vi "serial-read-mxp-board.vi"() -> ()   [LabVIEW 2018]
uses:
  bno055.ctl
  <vilib>/Rock Robotics/WPI/SerialPort/WPI_SerialPort.ctl
panel:
  out "BNO055":T1
  in  "stop":bool
  out "Read String":string
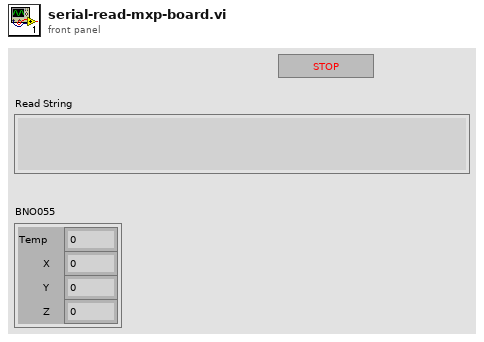
[diagram p1: front panel]
types:
  T1 = typedef "bno055.ctl" = cluster{"Temp":dbl, "X":dbl, "Y":dbl, "Z":dbl}
  T2 = typedef "WPI_SerialPort.ctl" = enum16{"Onboard RS-232", "MXP TTL", "USB 1", "USB 2"}
  T3 = typedef "WPI_SerialPortRef.ctl" = cluster{"DevStatus":errorcluster, "Serial Port Name":refnum<visa-resource-name>}
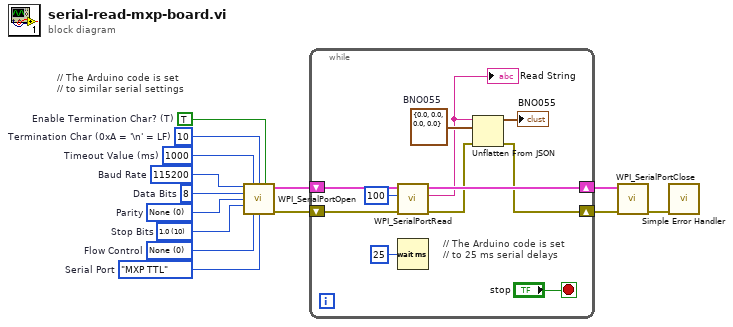
[diagram p0: block diagram]
diagram:
  w4 = WPI_SerialPort."MXP TTL"  # Serial Port
  w5 = u16 0 items=["None", "XON/XOFF", "RTS/CTS", "XON/XOFF & RTS/CTS", "DTR/DSR", "XON/XOFF & DTR/DSR"]  # Flow Control
  w6 = u16 10 items=["1.0"=10, "1.5"=15, "2.0"=20]  # Stop Bits
  w7 = u16 0 items=["None", "Odd", "Even", "Mark", "Space"]  # Parity
  w3 = u16 8  # Data Bits
  w8 = u32 115200  # Baud Rate
  w9 = u32 1000  # Timeout Value (ms)
  w10 = u8 10  # Termination Char (0xA = '\n' = LF)
  w11 = TRUE  # Enable Termination Char? (T)
  # "// The Arduino code is set \n// to similar serial settings"
  n1 = call <vilib>:"WPI_SerialPortOpen.vi"("Baud Rate"=w8, "Timeout Value (ms)"=w9, "Termination Char (0xA = '\\n' = LF)"=w10, "Enable Termination Char? (T)"=w11, "Data Bits"=w3, "Parity"=w7, "Stop Bits"=w6, "Flow Control"=w5, "Serial Port"=w4) -> ("SerialPortRef"=w2:T3, "error out"=w14:errorcluster)  [unwired: 5 in]
  n2 = while {
    shift-right: [w17] -> w13
    shift-left: w14 -> [w20]
    shift-right: [w25] -> w1
    shift-left: w2 -> [w21]
    stop <- "stop" stop-if-true
    w19 = T1 {"Temp"=0.0, "X"=0.0, "Y"=0.0, "Z"=0.0}  # BNO055
    # "// The Arduino code is set \n// to 25 ms serial delays"
    n3 = call <vilib>:"WPI_SerialPortRead.vi"("error in (no error)"=w20, "Num Bytes to Read"=u32 100, "SerialPortRef"=w21) -> ("error out"=w18:errorcluster, "Buffer"=w15:string, "SerialPortRef"=w25:T3)  [unwired: 6 in]
    "Read String" <- w15
    n4 = Wait (ms)(milliseconds to wait=u32 25) -> ()  [unwired: 1 out]
    n5 = Unflatten From JSON(JSON string=w15, type and defaults=w19, error in (no error)=w18) -> (value=→"BNO055":T1, error out=w17:errorcluster)  [unwired: 4 in]
  }
  n6 = call <vilib>:"WPI_SerialPortClose.vi"("error in (no error)"=w13, "SerialPortRef"=w1) -> ("error out"=w12:errorcluster)  [unwired: 9 in]
  n7 = call <vilib>:"Simple Error Handler.vi"("error in (no error)"=w12) -> ()  [unwired: 4 in, 5 out]
